vi "gfitsio-malloc-parameters-for-image-read.vi"(9 "inc":i32[](array[numeric]), 10 "lpixel":i32[](array[numeric]), 11 "fpixel":i32[](array[numeric])) -> (3 "image dimensions":i32[](array[numeric]))   [LabVIEW 2019, in "gfitsio.lvlib"]
uses:
  gfitsio.lvlib
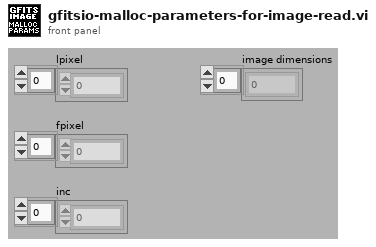
[diagram p1: front panel]
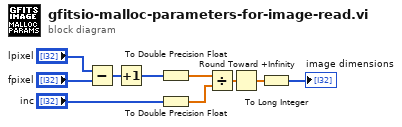
[diagram p0: block diagram]
diagram:
  n1 = Subtract(x="lpixel", y="fpixel") -> (x-y=w6:i32[])
  n2 = Increment(x=w6) -> (x+1=w7:i32[])
  n3 = To Double Precision Float(number=w7) -> (double precision float=w2:dbl[])
  n4 = To Double Precision Float(number="inc") -> (double precision float=w1:dbl[])
  n5 = Divide(x=w2, y=w1) -> (x/y=w5:dbl[])
  n6 = Round Toward +Infinity(x=w5) -> (ceil(x): smallest int >= x=w4:dbl[])
  n7 = To Long Integer(number=w4) -> (32bit integer=→"image dimensions":i32[])
